vi "ROI to line length.vi"(10 "ROI":T1) -> (2 "Length (pix)":i32)   [LabVIEW 2013]
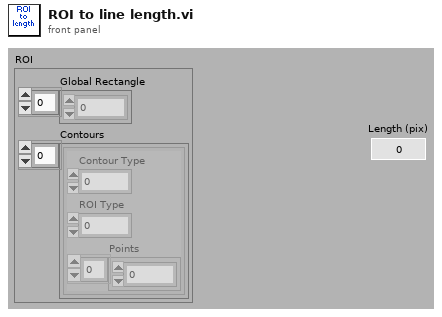
[diagram p1: front panel]
types:
  T1 = cluster{"Global Rectangle":i32[], "Contours":cluster{"Contour Type":u32, "ROI Type":u32, "Points":i32[]}[]}
  T2 = typedef "IMAQ Line" = cluster{"Start X":i32, "Start Y":i32, "End X":i32, "End Y":i32}
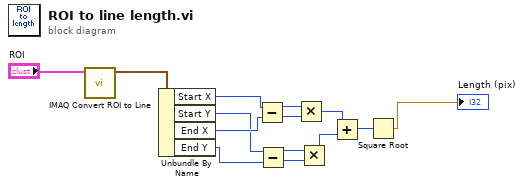
[diagram p0: block diagram]
diagram:
  n1 = call "IMAQ Convert ROI to Line"("ROI Descriptor"="ROI") -> ("Line"=w11:T2)  [unwired: 8 in, 1 out]
  n2 = Unbundle By Name(w11) -> ("Start X"=w7:i32, "Start Y"=w5:i32, "End X"=w6:i32, "End Y"=w4:i32)
  n3 = Subtract(x=w7, y=w6) -> (x-y=w10:i32)
  n4 = Subtract(x=w5, y=w4) -> (x-y=w9:i32)
  n5 = Multiply(x=w10, y=w10) -> (x*y=w3:i32)
  n6 = Multiply(x=w9, y=w9) -> (x*y=w2:i32)
  n7 = Add(x=w3, y=w2) -> (x+y=w8:i32)
  n8 = Square Root(x=w8) -> (sqrt(x)=→"Length (pix)":dbl)
